vi "chartsheet set footer lv.vi"(8 "error in (no error)":errorcluster, 10 "footer":string, 11 "chartsheet":u32) -> (0 "error out":errorcluster, 3 "function return":u32(ring))   [LabVIEW 2015, in "xlsxwriter.lvlib"]
doc: "lxw_error chartsheet_set_footer_lv(lxw_chartsheet chartsheet, const char *footer);"
uses:
  xlsxwriter.lvlib
  xlsxwriter.dll
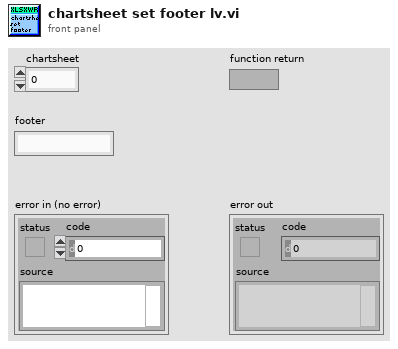
[diagram p1: front panel]
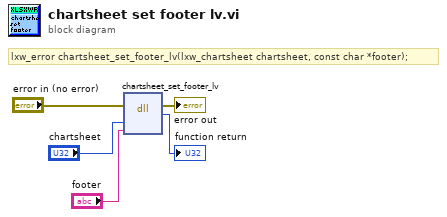
[diagram p0: block diagram]
diagram:
  # "lxw_error chartsheet_set_footer_lv(lxw_chartsheet chartsheet, const char *footer);"
  n1 = dll-call lib="C:/Users/WDAGUtilityAccount/Desktop/lv_vis_added_cell/xlsxwriter.*" fn="chartsheet_set_footer_lv"(error in="error in (no error)", "chartsheet"="chartsheet", "footer"="footer") -> (error out=→"error out":errorcluster, →"function return":u32)  [unwired: 4 in, 1 out]
